vi "Clear sound buffer.vi"(8 "error in (no error)":errorcluster, 11 "task ID":T1 format="%.0x") -> (0 "error out":errorcluster)   [LabVIEW 2019]
uses:
  <vilib>/sound2/lvsound2.llb/Sound Output Task ID.ctl
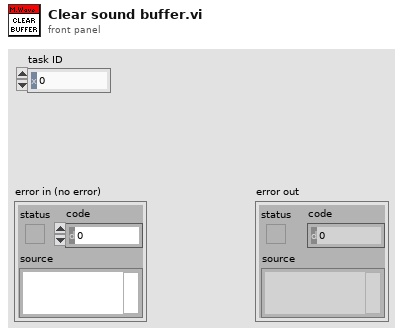
[diagram p1: front panel]
types:
  T1 = typedef "Sound Output Task ID.ctl" = u32
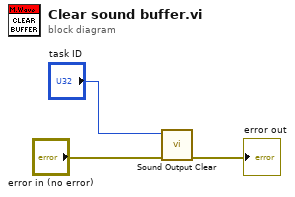
[diagram p0: block diagram]
diagram:
  n1 = call <vilib>:"Sound Output Clear.vi"("error in (no error)"="error in (no error)", "task ID"="task ID") -> ("error out"=→"error out":errorcluster)  [unwired: 9 in]
